vi "Average Waveforms Array.vi"(7 "Transpose?":bool, 8 "Error In":errorcluster, 9 "Waveforms In":waveform(dbl)[][](array[waveform])) -> (0 "Error Out":errorcluster, 1 "Averaged Waveforms":waveform(dbl)[](array[waveform]))   [LabVIEW 2019]
uses:
  <vilib>/Analysis/baseanly.llb/Mean (DBL).vi
  <vilib>/Analysis/NI_AALBase.lvlib
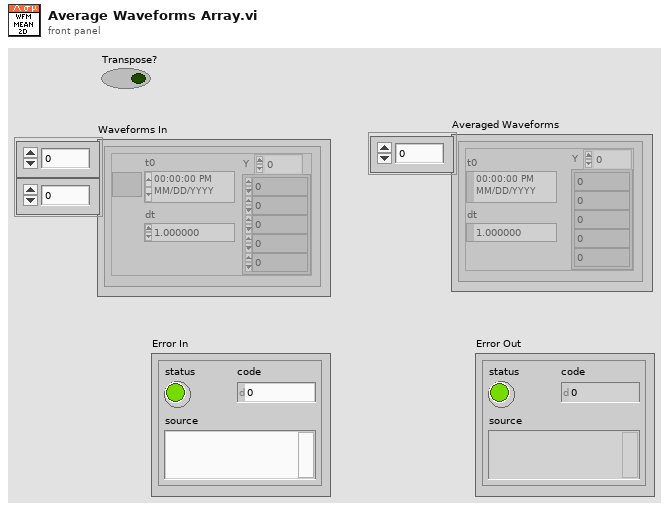
[diagram p1: front panel]
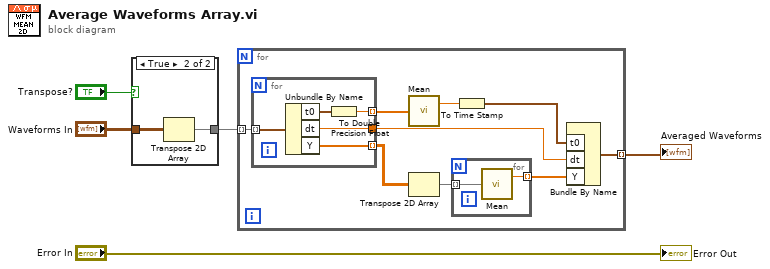
[diagram p0: block diagram]
diagram:
  n1 = case shown="True" "Transpose?" {
    tunnel: "Waveforms In" -> [w6 w8]
    tunnel: [w6 w7] -> w2
    frame False {
    }
    frame True {
      n2 = Transpose 2D Array(2D array=w8) -> (transposed array=w7:waveform(dbl)[][])
    }
  }
  n3 = for {
    tunnel: w2 -> [w15] mode=indexing
    tunnel: [w10] -> w4 mode=indexing
    n4 = for {
      tunnel: w15 -> [w22] mode=indexing
      tunnel: [w21] -> w9
      tunnel: [w20] -> w14 mode=indexing
      tunnel: [w18] -> w12 mode=indexing
      n5 = Unbundle By Name(w22) -> ("t0"=w19:timestamp, "dt"=w21:dbl, "Y"=w20:dbl[])
      n6 = To Double Precision Float(number=w19) -> (double precision float=w18:dbl)
    }
    n7 = call-poly <vilib>:"Mean.vi"("X"=w12) -> ("mean"=w13:dbl)  [unwired: 1 out]
    n8 = Transpose 2D Array(2D array=w14) -> (transposed array=w16:dbl[][])
    n9 = for {
      tunnel: w16 -> [w24] mode=indexing
      tunnel: [w23] -> w17 mode=indexing
      n10 = call-poly <vilib>:"Mean.vi"("X"=w24) -> ("mean"=w23:dbl)  [unwired: 1 out]
    }
    n11 = To Time Stamp(1:w13) -> (0:w11:timestamp)
    n12 = Bundle By Name("t0"=w11, "dt"=w9, "Y"=w17) -> (w10:waveform(dbl))  [unwired: 1 in]
  }
  "Averaged Waveforms" <- w4
  "Error Out" <- "Error In"
